vi "getScriptPath.vi"(8 "error in (no error)":errorcluster, 11 "Point.lvclass in":refnum<class "Point.lvclass">) -> (0 "error out":errorcluster, 2 "dpScriptPath":path, 3 "Point.lvclass out":refnum<class "Point.lvclass">)   [LabVIEW 2011, in "Tools.lvlib" / "Sequencing.lvlib" / "Point.lvclass"]
uses:
  Point.lvclass
  Point.lvclass/Point.ctl
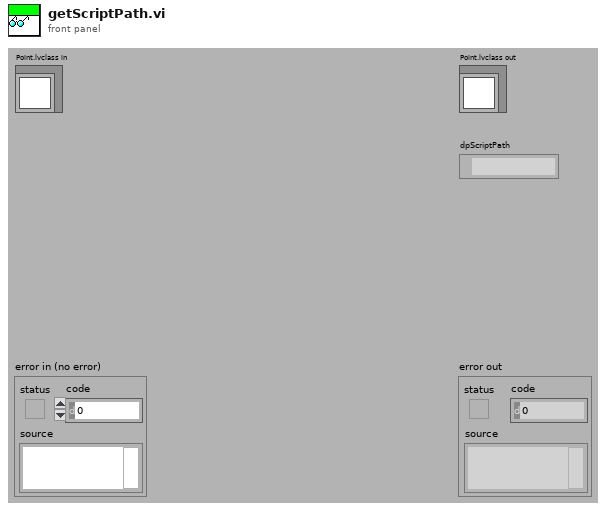
[diagram p1: front panel]
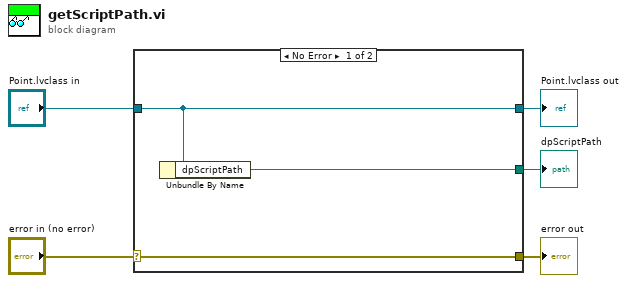
[diagram p0: block diagram]
diagram:
  n1 = case shown="No Error" "error in (no error)" {
    selector: "error in (no error)" -> [w8 w9]
    tunnel: [w8 w9] -> w4
    tunnel: [w7 w10] -> w2
    tunnel: "Point.lvclass in" -> [w7 w10]
    tunnel: [w6 _] -> w1
    frame No Error {
      n2 = Unbundle By Name(w7) -> ("dpScriptPath"=w6:path)
    }
    frame Error {
    }
  }
  "error out" <- w4
  "Point.lvclass out" <- w2
  "dpScriptPath" <- w1
